vi "Unary routeguide_RouteGuide_GetFeature.vi"(8 "error in":errorcluster, 9 "contextId":T1, 10 "Request Data":T3, 11 "gRPC ID":T1) -> (0 "error out":errorcluster, 2 "Response Data":T2, 3 "gRPC ID out":T1)   [LabVIEW 2019, in "route_guide_client.lvlib"]
uses:
  route_guide_client.lvlib
  RPC Messages/routeguide_Point.ctl
  RPC Messages/routeguide_Feature.ctl
  1d5000e3-7ad3-439f-848e-744714f1e255.vi
  <vilib>/gRPC/LabVIEW gRPC Library/Shared/grpcId.ctl
  <vilib>/gRPC/LabVIEW gRPC Library/grpc-lvsupport-release.lvlib
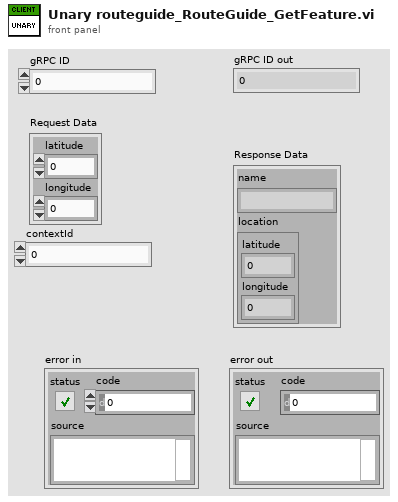
[diagram p1: front panel]
types:
  T1 = typedef "grpc-lvsupport-release.lvlib/grpcId.ctl" = u64
  T2 = typedef "route_guide_client.lvlib/routeguide_Feature.ctl" = cluster{"name":string, "location":T3}
  T3 = typedef "route_guide_client.lvlib/routeguide_Point.ctl" = cluster{"latitude":i32, "longitude":i32}
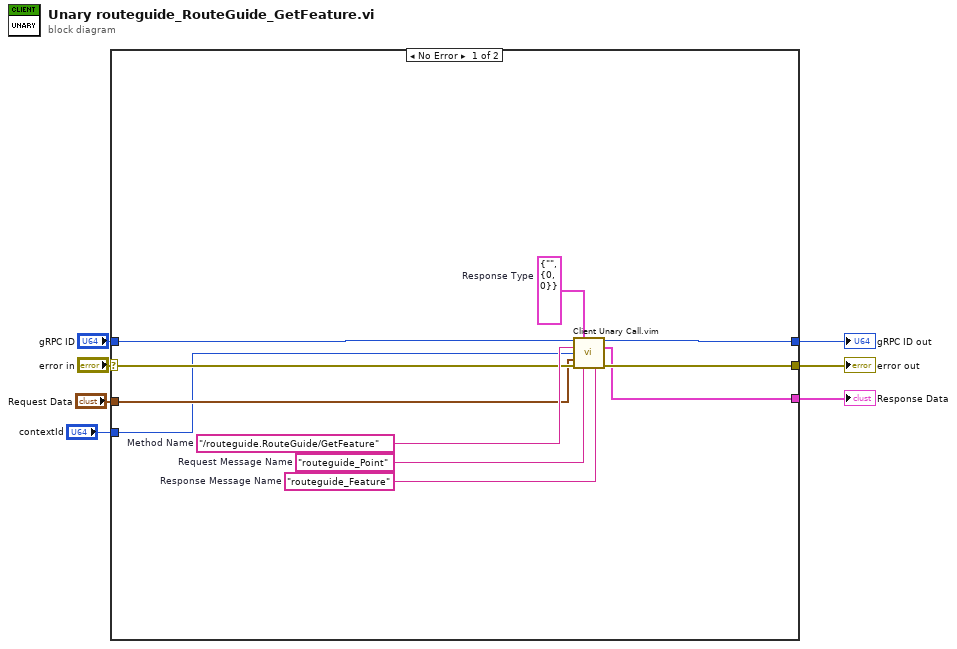
[diagram p0: block diagram]
diagram:
  n1 = case shown="No Error" "error in" {
    selector: "error in" -> [w14 w19]
    tunnel: [w13 w19] -> w6
    tunnel: "gRPC ID" -> [w12 w20]
    tunnel: [w11 w20] -> w4
    tunnel: "Request Data" -> [w10 _]
    tunnel: [w9 _] -> w2
    tunnel: "contextId" -> [w8 _]
    frame No Error {
      w15 = "routeguide_Feature"  # Response Message Name
      w16 = "routeguide_Point"  # Request Message Name
      w17 = T2 {"name"="", "location"={"latitude"=0, "longitude"=0}}  # Response Type
      w18 = "/routeguide.RouteGuide/GetFeature"  # Method Name
      n2 = call "Client Unary Call.vim"("ClientID in"=w12, "Response Type"=w17, "Method Name"=w18, "contextId"=w8, "Request Data"=w10, "error in"=w14, "Request Message Name"=w16, "Response Message Name"=w15) -> ("ClientID out"=w11:u64, "Response Data"=w9:T2, "error out"=w13:errorcluster)  [unwired: 5 in]
    }
    frame Error {
    }
  }
  "error out" <- w6
  "gRPC ID out" <- w4
  "Response Data" <- w2
